vi "TestReceiveMessage.vi"() -> ()   [LabVIEW 2016]
uses:
  CAN_Info.ctl
  MessageInfo.ctl
  SendMsgInfo.ctl
panel:
  out "布尔":bool=TRUE
  out "tsapp_receive_can_messageList 2":T1[](array[typedef])
  in  "错误输入（无错误） 2":errorcluster caption="错误输入（无错误）"
  out "tsapp_receive_can_message":bool
  out "错误输出 2":errorcluster caption="错误输出"
  out "tsapp_clear_can_receive_buffers":i32
  out "tsapp_connect":i32
  out "ConnectSeccessfully 2":bool
  out "SetSuccessfully":bool
  out "错误输出":errorcluster
  out "InitializationInformation_Out":T2 {"LIN使用通道数" max=5; "CAN使用通道数" max=5}
  out "tsapp_disconnect":i32
  out "DisConnectSeccessfully":bool
  in  "错误输入（无错误）":errorcluster
  out "initialize_lib_tsmaster":i32
  out "initialize_lib_tsmaster_ok":bool
  out "InitializationInformation":T2 {"LIN使用通道数" max=5; "CAN使用通道数" max=5}
  out "应用程序名":string
  out "funtcion_return":i32
  out "帧数":i32(graph)
  in  "停止":bool
  out "时间":u32(graph)
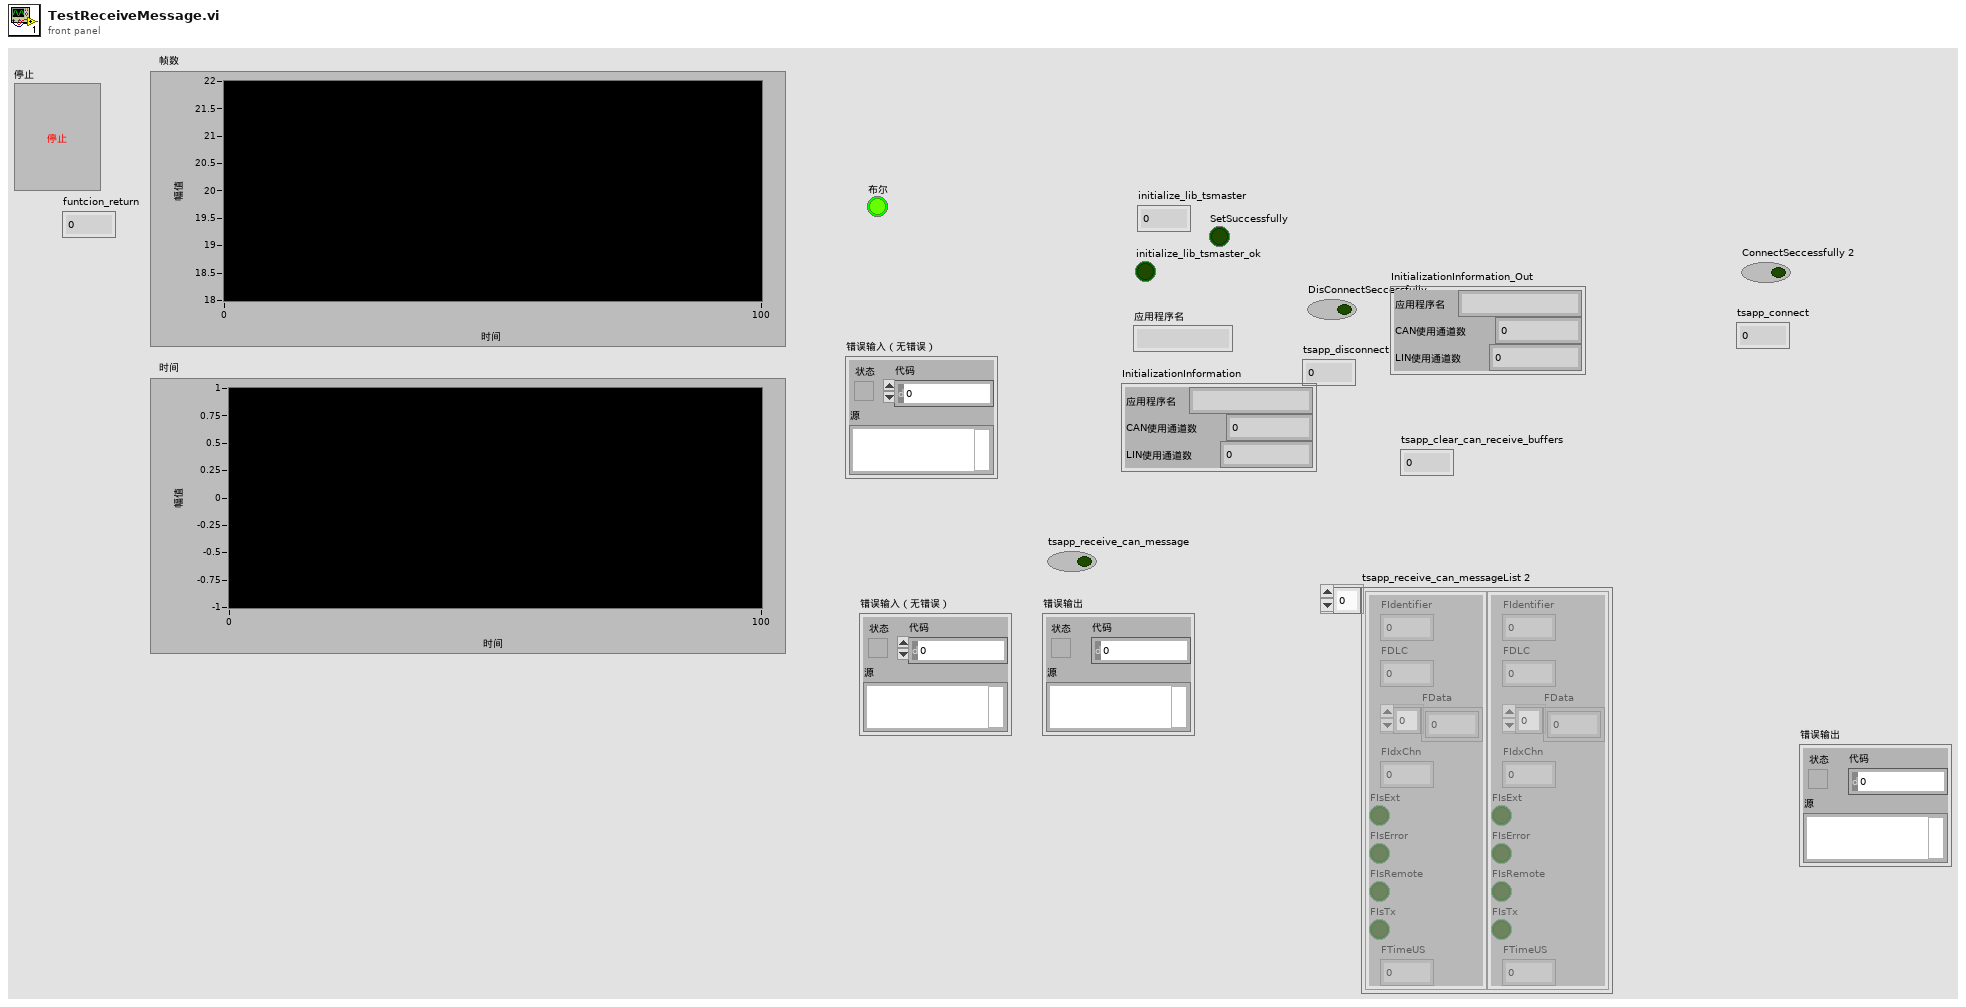
[diagram p1: front panel]
types:
  T1 = typedef "MessageInfo.ctl" = cluster{"FIdentifier":i32, "FDLC":u8, "FData":u8[], "FIdxChn":u8, "FIsExt":bool, "FIsError":bool, "FIsRemote":bool, "FIsTx":bool, "FTimeUS":u64}
  T2 = typedef "CAN_Info.ctl" = cluster{"应用程序名":string, "CAN使用通道数":u8, "LIN使用通道数":u8}
  T3 = typedef "SendMsgInfo.ctl" = cluster{"FIdxChn":u8, "FProperties":u8, "FDLC":u8, "FReserved":u8, "FIdentifier":i32, "FTimeUS":u64, "Data0":u8, "Data1":u8, "Data2":u8, "Data3":u8, "Data4":u8, "Data5":u8, "Data6":u8, "Data7":u8}
  T4 = typedef "TCANProperty.ctl" = cluster{"istx":bool, "remoteframe":bool, "extframe":bool, "tbd1":bool, "tbd2":bool, "tbd3":bool, "tbd4":bool, "iserrorframe":bool}
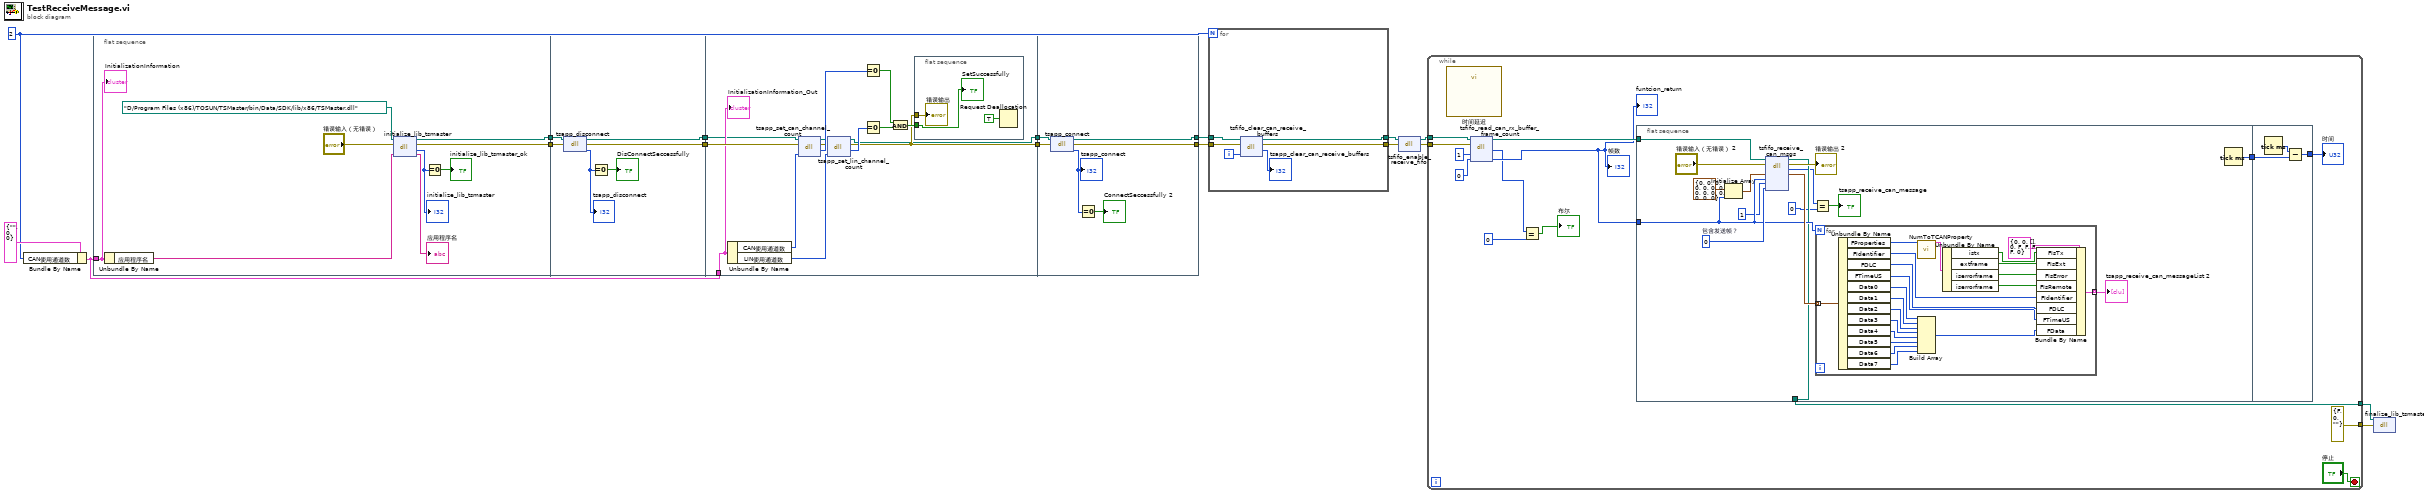
[diagram p0: block diagram]
diagram:
  w16 = u8 2 ("CAN使用通道数")
  n1 = Bundle By Name(cluster=T2 {"应用程序名"="", "CAN使用通道数"=0, "LIN使用通道数"=0} ("初始化CAN通道"), "CAN使用通道数"=w16) -> (w10:T2)
  n2 = flat-sequence {
    tunnel: w10 -> [w21]
    tunnel: [w20] -> w12
    tunnel: [w18] -> w7
    tunnel: w12 -> [w30]
    tunnel: [w29] -> w11
    tunnel: w7 -> [w28]
    tunnel: [w27] -> w6
    tunnel: w11 -> [w37]
    tunnel: w10 -> [w36]
    tunnel: [w38] -> w9
    tunnel: w6 -> [w35]
    tunnel: [w33] -> w5
    tunnel: w9 -> [w52]
    tunnel: [w53] -> w8
    tunnel: w5 -> [w51]
    tunnel: [w50] -> w4
    frame #0 {
      n3 = Unbundle By Name(w21) -> ("应用程序名"=w26:string)
      n4 = dll-call lib="D:/Program Files (x86)/TOSUN/TSMaster/bin/Data/SDK/lib/x86/TSMaster.dll" fn="initialize_lib_tsmaster"(path in=path "D:/Program Files (x86)/TOSUN/TSMaster/bin/Data/SDK/lib/x86/TSMaster.dll" ("路径输入"), error in="错误输入（无错误）", "AAppName"=w26) -> (path out=w18:path, error out=w20:errorcluster, "initialize_lib_tsmaster"=w24:i32, "AAppName"=→"应用程序名":string)  [unwired: 1 in]
      "initialize_lib_tsmaster" <- w24
      n5 = Equal To 0?(x=w24) -> (x = 0?=→"initialize_lib_tsmaster_ok":bool)
      "InitializationInformation" <- w21
    }
    frame #1 {
      n6 = dll-call lib="D:/Program Files (x86)/TOSUN/TSMaster/bin/Data/SDK/lib/x86/TSMaster.dll" fn="tsapp_disconnect"(path in=w28, error in=w30) -> (path out=w27:path, error out=w29:errorcluster, "tsapp_disconnect"=w31:i32)  [unwired: 1 in]
      "tsapp_disconnect" <- w31
      n7 = Equal To 0?(x=w31) -> (x = 0?=→"DisConnectSeccessfully":bool)
    }
    frame #2 {
      n8 = Unbundle By Name(w36) -> ("CAN使用通道数"=w41:u8, "LIN使用通道数"=w42:u8)
      n9 = dll-call lib="PTH2Oabs D\n26-LV_proj69-调用TSMaster2021041569-调用TSMasterTSMaster.dll" fn="tsapp_set_can_channel_count"(path in=w35, error in=w37, "ACount"=w41) -> (path out=w34:path, error out=w39:errorcluster, "tsapp_set_can_channel_count"=w45:i32)  [unwired: 2 in]
      n10 = dll-call lib="PTH2Oabs D\n26-LV_proj69-调用TSMaster2021041569-调用TSMasterTSMaster.dll" fn="tsapp_set_lin_channel_count"(path in=w34, error in=w39, "ACount"=w42) -> (path out=w33:path, error out=w38:errorcluster, "tsapp_set_can_channel_count"=w40:i32)  [unwired: 2 in]
      n11 = Equal To 0?(x=w45) -> (x = 0?=w43:bool)
      n12 = Equal To 0?(x=w40) -> (x = 0?=w44:bool)
      n13 = And(x=w43, y=w44) -> (x .and. y?=w46:bool)
      n14 = flat-sequence {
        tunnel: w46 -> [w49]
        tunnel: w38 -> [w48]
        frame #0 {
          n15 = Request Deallocation(TRUE ("标志")) -> ()
          "SetSuccessfully" <- w49
          "错误输出" <- w48
        }
      }
      "InitializationInformation_Out" <- w36
    }
    frame #3 {
      n16 = dll-call lib="PTH2Oabs D\n26-LV_proj69-调用TSMaster2021041569-调用TSMasterTSMaster.dll" fn="tsapp_connect"(path in=w51, error in=w52) -> (path out=w50:path, error out=w53:errorcluster, "tsapp_connect"=w55:i32)  [unwired: 1 in]
      "tsapp_connect" <- w55
      n17 = Equal To 0?(x=w55) -> (x = 0?=→"ConnectSeccessfully 2":bool)
    }
  }
  n18 = for {
    N: w16 -> [_]
    tunnel: w8 -> [w59]
    tunnel: [w58] -> w14
    tunnel: w4 -> [w57]
    tunnel: [w56] -> w3
    i -> [w60]
    n19 = dll-call lib="PTH2Oabs D\n26-LV_proj69-调用TSMaster2021041569-调用TSMasterTSMaster.dll" fn="tsfifo_clear_can_receive_buffers"(path in=w57, error in=w59, "AChn"=w60) -> (path out=w56:path, error out=w58:errorcluster, "tsapp_clear_can_receive_buffers"=→"tsapp_clear_can_receive_buffers":i32)  [unwired: 2 in]
  }
  n20 = dll-call lib="D:/Program Files (x86)/TOSUN/TSMaster/bin/Data/SDK/lib/x86/TSMaster.dll" fn="tsfifo_enable_receive_fifo"(path in=w3, error in=w14) -> (path out=w2:path, error out=w13:errorcluster)  [unwired: 2 in]
  n21 = while {
    tunnel: w13 -> [w69]
    tunnel: [errorcluster {"status"=FALSE, "code"=0, "source"=""} ("错误输入（无错误）")] -> w15
    tunnel: w2 -> [w68]
    tunnel: [w66] -> w1
    stop <- "停止" stop-if-true
    n22 = call "时间延迟"() -> ()  [unwired: 11 in, 1 out]
    n23 = dll-call lib="D:/Program Files (x86)/TOSUN/TSMaster/bin/Data/SDK/lib/x86/TSMaster.dll" fn="tsfifo_read_can_rx_buffer_frame_count"(path in=w68, error in=w69, "AChn"=1, "AFrameCount"=0 ("参数2")) -> (path out=w67:path, "funtcion_return"=w64:i32, "AFrameCount"=w65:i32)  [unwired: 2 in, 1 out]
    "帧数" <- w65
    "funtcion_return" <- w65
    n24 = Equal?(x=w64, y=0) -> (x = y?=→"布尔":bool)
    n25 = flat-sequence {
      tunnel: w65 -> [w81]
      tunnel: [w90] -> w73
      tunnel: w67 -> [w79]
      tunnel: [w78] -> w66
      tunnel: [w114] -> w74
      tunnel: w73 -> [w112]
      frame #0 {
        w84 = u8 0  # 包含发送帧？
        n26 = Initialize Array(T3 {"FIdxChn"=0, "FProperties"=0, "FDLC"=0, "FReserved"=0, "FIdentifier"=0, "FTimeUS"=0, "Data0"=0, "Data1"=0, "Data2"=0, "Data3"=0, "Data4"=0, "Data5"=0, "Data6"=0, "Data7"=0} ("SendMsgInfo"), w81) -> (w88:T3[])
        n27 = dll-call lib="D:/Program Files (x86)/TOSUN/TSMaster/bin/Data/SDK/lib/x86/TSMaster.dll" fn="tsfifo_receive_can_msgs"(path in=w79, error in="错误输入（无错误） 2", "ACANBuffers"=w88, "ACANBufferSize"=w81, "AChn"=1 ("AAppChannel输入"), "ARxTx"=w84) -> (path out=w78:path, error out=→"错误输出 2":errorcluster, "tsapp_receive_can_msgs"=w77:i32, "ACANBuffers"=w86:T3[])  [unwired: 4 in]
        n28 = Equal?(x=w77, y=0) -> (x = y?=→"tsapp_receive_can_message":bool)
        n29 = for {
          N: w81 -> [_]
          tunnel: [w111] -> w89 mode=indexing
          tunnel: w86 -> [w109] mode=indexing
          n30 = Unbundle By Name(w109) -> ("FProperties"=w108:u8, "FIdentifier"=w102:i32, "FDLC"=w101:u8, "FTimeUS"=w100:u64, "Data0"=w99:u8, "Data1"=w98:u8, "Data2"=w97:u8, "Data3"=w96:u8, "Data4"=w95:u8, "Data5"=w94:u8, "Data6"=w93:u8, "Data7"=w92:u8)
          n31 = call "NumToTCANProperty.vi"("TCANPropertyNum"=w108) -> ("TCANProperty"=w107:T4)  [unwired: 10 in]
          n32 = Build Array(w99, w98, w97, w96, w95, w94, w93, w92) -> (w91:u8[])
          n33 = Unbundle By Name(w107) -> ("istx"=w106:bool, "extframe"=w105:bool, "iserrorframe"=w104:bool, "iserrorframe"=w103:bool)
          n34 = Bundle By Name(cluster=T1 {"FIdentifier"=0, "FDLC"=0, "FData"=[], "FIdxChn"=0, "FIsExt"=FALSE, "FIsError"=FALSE, "FIsRemote"=FALSE, "FIsTx"=FALSE, "FTimeUS"=0} ("Receive message"), "FIsTx"=w106, "FIsExt"=w105, "FIsError"=w104, "FIsRemote"=w103, "FIdentifier"=w102, "FDLC"=w101, "FTimeUS"=w100, "FData"=w91) -> (w111:T1)
        }
        "tsapp_receive_can_messageList 2" <- w89
        n35 = Tick Count (ms)() -> (millisecond timer value=w90:u32)
      }
      frame #1 {
        n36 = Tick Count (ms)() -> (millisecond timer value=w113:u32)
        n37 = Subtract(x=w113, y=w112) -> (x-y=w114:u32)
      }
    }
    "时间" <- w74
  }
  n38 = dll-call lib="PTH2habs D\n26-LV_proj69-调用TSMaster2021041569-调用TSMasterTSMaster_LV2010_ReleaseTSMaster.dll" fn="finalize_lib_tsmaster"(path in=w1, error in=w15) -> ()  [unwired: 2 in, 2 out]
